vi "LcTfCal.vi"() -> ()   [LabVIEW 2013]
panel:
  in  "stop":bool
  out "Plot 1":dynamicdata(graph)
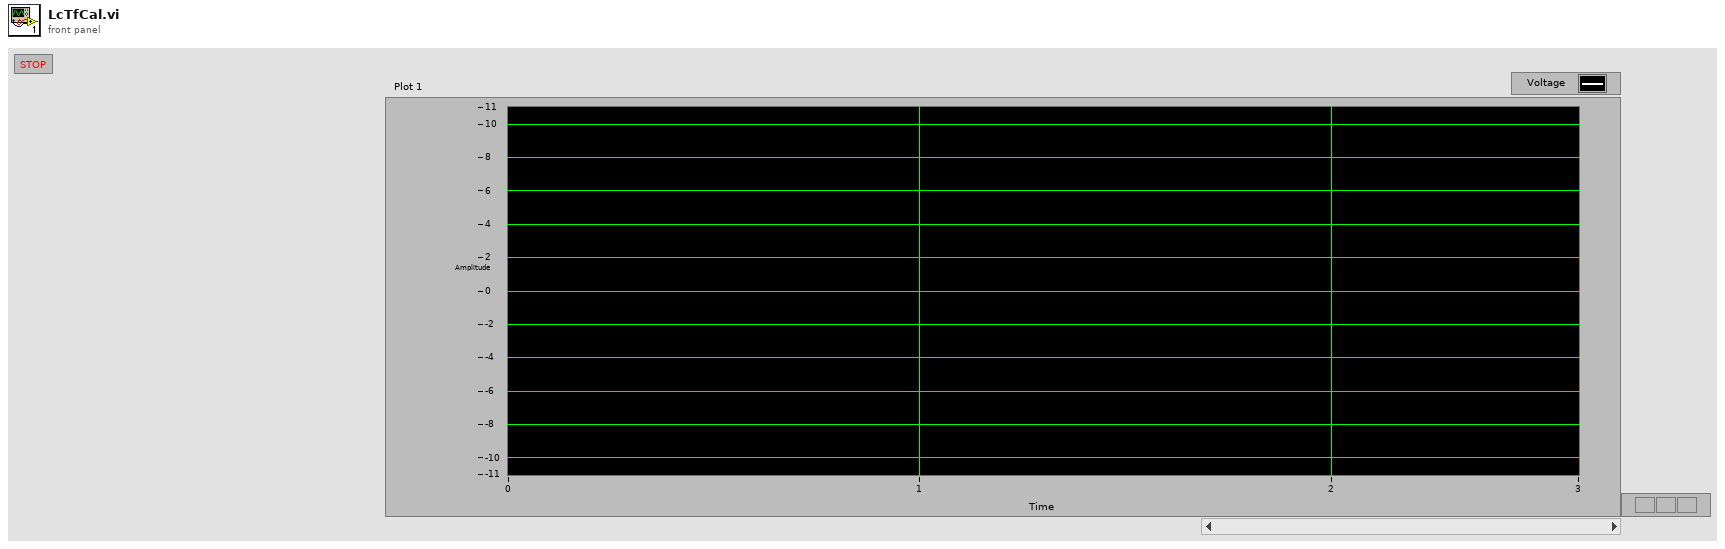
[diagram p1: front panel]
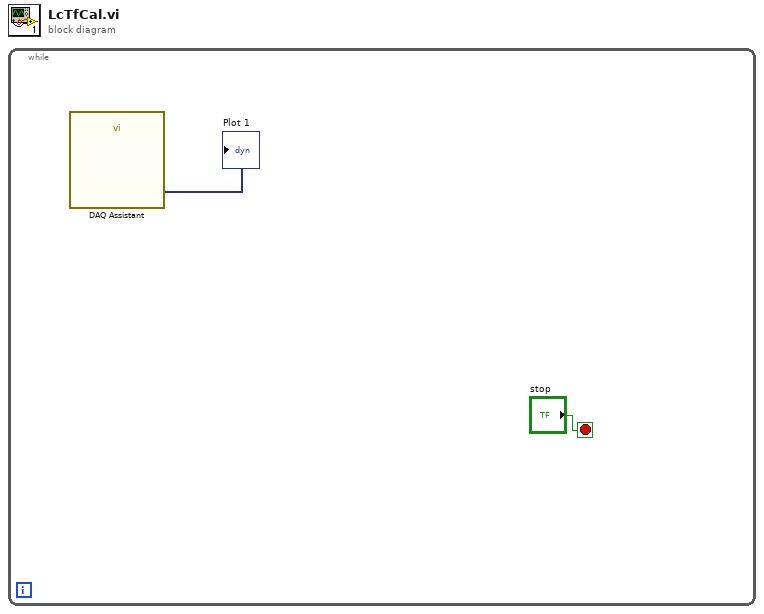
[diagram p0: block diagram]
diagram:
  n1 = while {
    stop <- "stop" stop-if-true
    n2 = call "DAQ Assistant"() -> ("data"=→"Plot 1":dynamicdata)  [unwired: 16 in, 3 out]
  }
